vi "c ctre phoenixpro Request Control Strict Follower.vi"(6 "MasterID":i32, 7 "cancelOtherRequests":bool, 8 "error in (no error)":errorcluster, 9 "updateTime":dbl, 10 "ecuEncoding":u32, 11 "canbus":string) -> (0 "error out":errorcluster, 3 "function return":i32)   [LabVIEW 2020, in "CTRE_PhoenixTools.lvlib"]
doc: "CTREXPORT int c_ctre_phoenixpro_RequestControlStrictFollower(const char *canbus, uint32_t ecuEncoding, double updateTime, bool cancelOtherRequests, int MasterID);"
uses:
  CTRE_PhoenixTools.lvlib
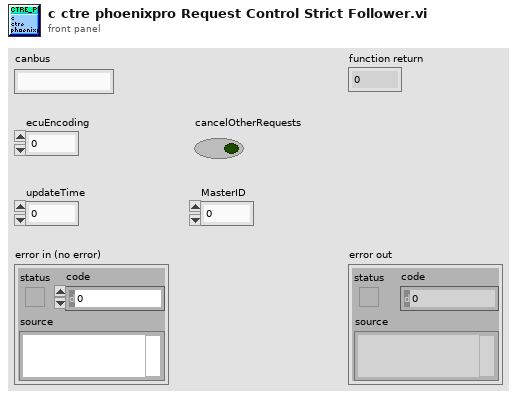
[diagram p1: front panel]
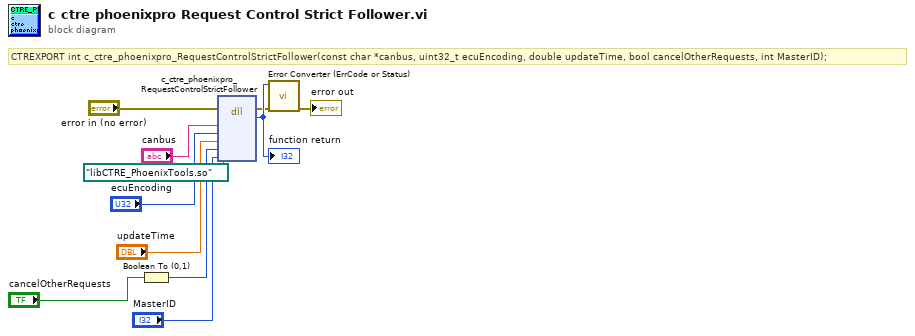
[diagram p0: block diagram]
diagram:
  # "CTREXPORT int c_ctre_phoenixpro_RequestControlStrictFollower(const char *canbus, uint32_t ecuEncoding, double updateTime, bool cancelOtherRequests, int MasterID);"
  n1 = Boolean To (0,1)(Boolean="cancelOtherRequests") -> (0, 1=w6:i16)
  n2 = dll-call lib="?" fn="c_ctre_phoenixpro_RequestControlStrictFollower"(path in=path "libCTRE_PhoenixTools.so", error in="error in (no error)", "canbus"="canbus", "ecuEncoding"="ecuEncoding", "updateTime"="updateTime", "cancelOtherRequests"=w6, "MasterID"="MasterID") -> (error out=w3:errorcluster, w11:i32)  [unwired: 6 in, 1 out]
  "function return" <- w11
  n3 = call "Error Converter (ErrCode or Status).vi"("error in (no error)"=w3, "error code"=w11) -> ("error out"=→"error out":errorcluster)  [unwired: 9 in]
